vi "Report Raw Data.vi"(9 "Data":T1={"Datetime"="DateTime", "User Name"="Barcode", "Running Model"="Operator_Name", "Barcode"="Operator_Name", "Barcode difusser"="Operator_Name"}, 10 "Sensor Data":T2={"Load Min(N)"="Load min(N)", "Load Max(N)"="Load max(N)", "Load(N) "="Load (N)", "Dist Min(mm)"="Dist min(mm)", "Dist Max(mm)"="Dist max(mm)", "Dist (mm)"="Dist (mm)", "Load Status"="Load Status", "Dist Status"="Dist Status"}, 11 "test":string[][](array[string])=[["1", "Light Box Ionization", "Pass"], ["2", "Light box Clamp", "Pass"], ["3", "Difusser Put on Light Box", "Pass"], ["4", "Photo Prism Put On LB", "Test In Progress"], ["5", "LCD Put On Light Box", ""], ["6", "Difusser Checking Position", ""], ["7", "Adesive Tap check Camera", ""], ["8", "LCD Placing Position", ""], ["9", "Camera check Adhesive Taps", ""], ["10", "LCD Display Rotating ", ""], ["11", "Camera Slide Unit", ""], ["12", "LCD Pressing Servo", ""], ["13", "LCD Pressing servo up", ""], ["14", "Camera Unit Rev", ""], ["15", "Fixture Slide Up", ""], ["16", "Light Box Unclamp", ""]]) -> (1 "Machine Status":bool, 2 "Data":string[](array[string]), 3 "Header":string[](array[string]))   [LabVIEW 2020]
uses:
  Galobal variable_TI.vi
panel:
  out "Array":bool[](array[boolean])
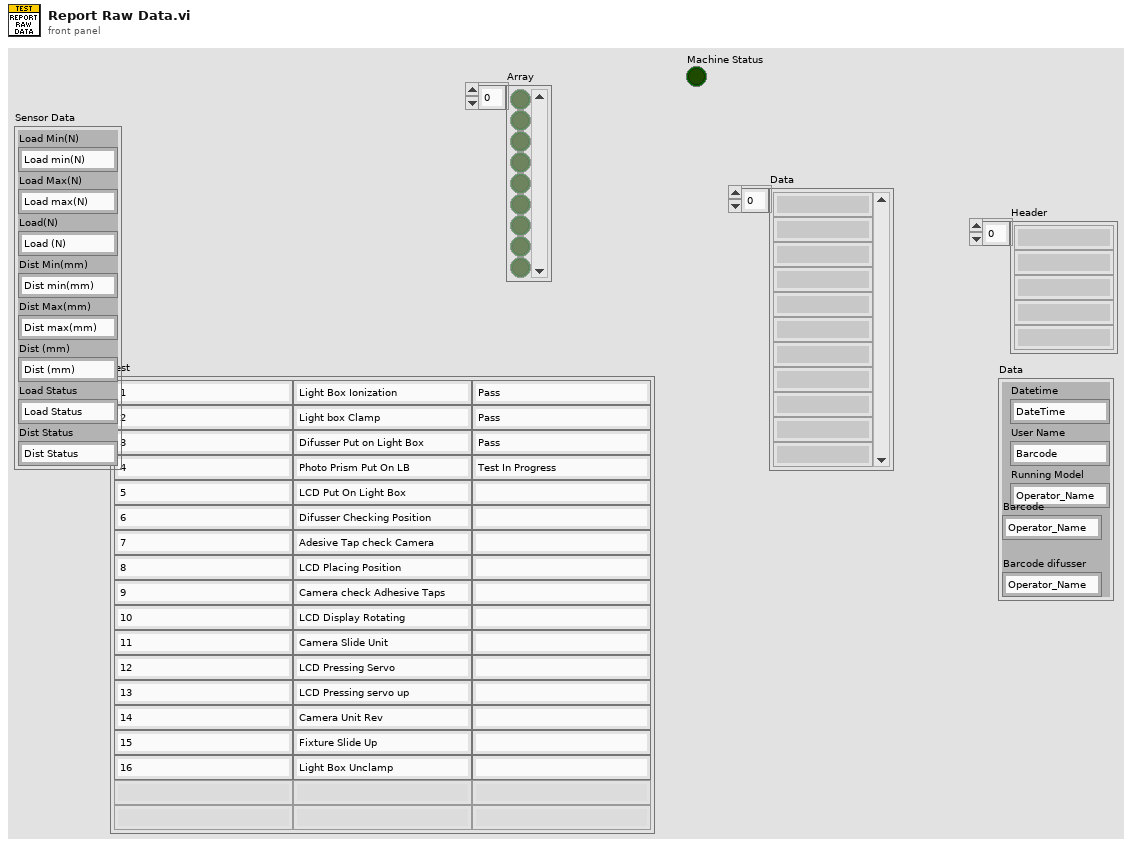
[diagram p1: front panel]
types:
  T1 = cluster{"Datetime":string, "User Name":string, "Running Model":string, "Barcode":string, "Barcode difusser":string}
  T2 = cluster{"Load Min(N)":string, "Load Max(N)":string, "Load(N) ":string, "Dist Min(mm)":string, "Dist Max(mm)":string, "Dist (mm)":string, "Load Status":string, "Dist Status":string}
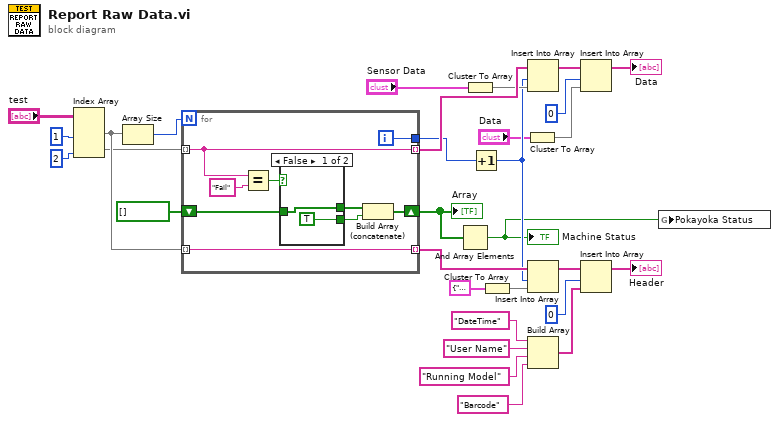
[diagram p0: block diagram]
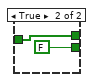
[diagram p2: hidden frame]
diagram:
  n1 = Index Array(array="test", index (col) #1=1 ("disabled index (col)"), index (col) #2=2 ("index (col)")) -> (element #1=w27:string[], element #2=w26:string[])  [unwired: 2 in]
  n2 = Array Size(array=w27) -> (size(s)=w4:i32)
  n3 = for {
    N: w4 -> [_]
    tunnel: w27 -> [w39] mode=indexing
    tunnel: w26 -> [w35] mode=indexing
    tunnel: [w39] -> w21 mode=indexing
    tunnel: [w35] -> w25 mode=indexing
    tunnel: [w38] -> w24
    shift-right: [w33] -> w2
    shift-left: bool[] [] -> [w32]
    i -> [w38]
    n4 = Equal?(x=w35, y="Fail") -> (x = y?=w36:bool)
    n5 = case shown="False" w36 {
      tunnel: [TRUE FALSE] -> w34
      tunnel: w32 -> [w41 w42]
      tunnel: [w41 w42] -> w31
      frame False {
      }
      frame True {
      }
    }
    n6 = Build Array (concatenate)(w31, w34) -> (w33:bool[])
  }
  "Array" <- w2
  n7 = And Array Elements(Boolean array=w2) -> (logical AND=w1:bool)
  "Machine Status" <- w1
  n8 = Cluster To Array(cluster="Sensor Data") -> (array=w23:string[])
  n9 = Increment(x=w24) -> (x+1=w20:i32)
  n10 = Cluster To Array(cluster=T2 {"Load Min(N)"="Load min(N)", "Load Max(N)"="Load max(N)", "Load(N) "="Load (N)", "Dist Min(mm)"="Load Status", "Dist Max(mm)"="Dist min(mm)", "Dist (mm)"="Dist max(mm)", "Load Status"="Dist (mm)", "Dist Status"="Dist Status"} ("Sensor Data 2")) -> (array=w19:string[])
  n11 = Cluster To Array(cluster="Data") -> (array=w7:string[])
  n12 = Insert Into Array(array=w25, index=w20, new element=w23) -> (w10:string[])
  n13 = Insert Into Array(array=w21, index=w20, new element=w19) -> (w13:string[])
  n14 = Build Array("DateTime", "User Name" ("element"), "Running Model" ("element"), "Barcode" ("element")) -> (w12:string[])
  n15 = Insert Into Array(array=w10, index=0, new element=w7) -> (→"Data":string[])
  n16 = Insert Into Array(array=w13, index=0, new element=w12) -> (→"Header":string[])
  n17 = global write "Galobal variable_TI.vi" "Pokayoka Status"(w1) -> ()
